vi "Agilent 34970 Reset Known State.vi"(8 "Error In":errorcluster, 11 "VISA Refnum in":refnum<visa-resource-name>) -> (0 "Error Out":errorcluster)   [LabVIEW 2019]
uses:
  Agilent 34970.lvlib
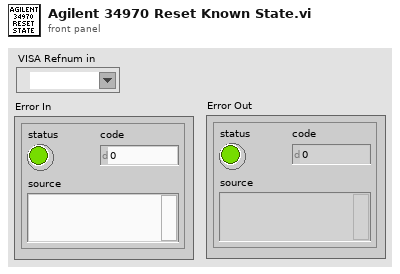
[diagram p1: front panel]
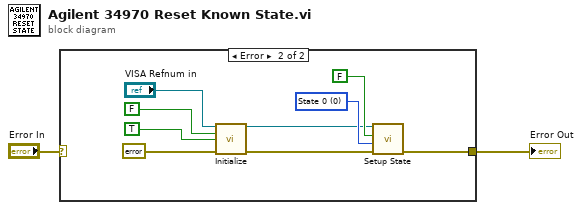
[diagram p0: block diagram]
diagram:
  n1 = case shown="Error" "Error In" {
    selector: "Error In" -> [w3 _]
    tunnel: [w3 w4] -> w2
    frame No Error {
    }
    frame Error {
      w11 = u16 0 items=["State 0", "State 1", "State 2", "State 3", "State 4", "State 5", "Preset State"] ("Setup State (6:Preset)")
      n2 = call "Initialize.vi"("VISA Resource Name"="VISA Refnum in", "ID Query (T: Check)"=FALSE, "Reset (T: Reset)"=TRUE, "error in (no error)"=errorcluster {"status"=FALSE, "code"=0, "source"=""}) -> ("VISA Resource Name Out"=w9:refnum<visa-resource-name>, "error out"=w8:errorcluster)  [unwired: 10 in]
      n3 = call "Setup State.vi"("error in (no error)"=w8, "Setup State (6:Preset)"=w11, "Recall/Save (F=Recall)"=FALSE, "VISA Resource Name"=w9) -> ("error out"=w4:errorcluster)  [unwired: 6 in, 1 out]
    }
  }
  "Error Out" <- w2
